vi "EMV Check All History to Cold Water Supply Temp.vi"(4 "T7_DELTA_FLOW_THRESHOLD":dbl, 6 "Cold Water Supply Temperature":dbl, 8 "error in (no error)":errorcluster, 11 "Current T7 Temperatures":dbl[](array[numeric])) -> (0 "error out":errorcluster, 5 "All History Is Near Supply Temp (T) = Flowing":bool)   [LabVIEW 2020]
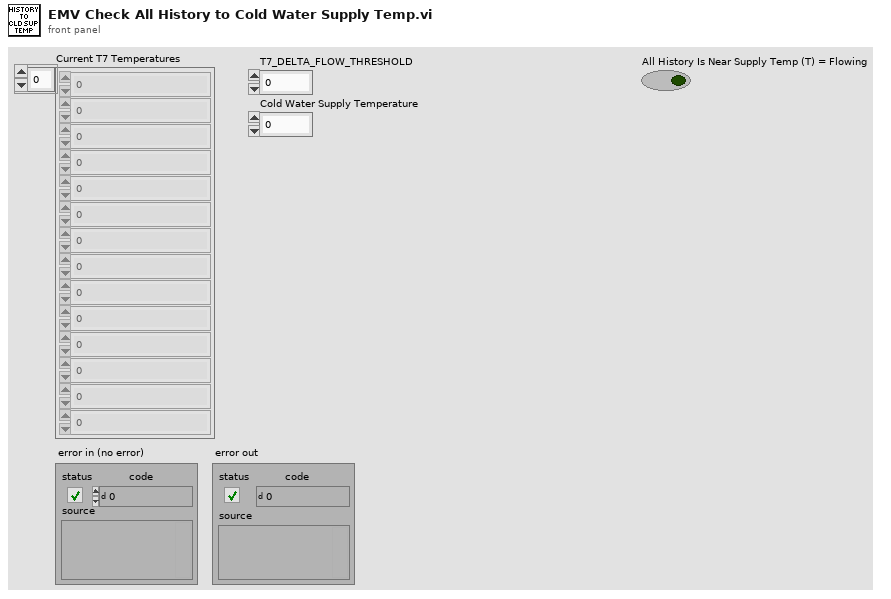
[diagram p1: front panel]
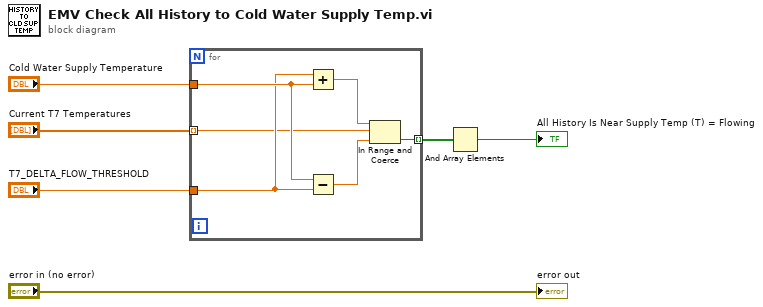
[diagram p0: block diagram]
diagram:
  n1 = for {
    tunnel: "Cold Water Supply Temperature" -> [w11]
    tunnel: "T7_DELTA_FLOW_THRESHOLD" -> [w10]
    tunnel: "Current T7 Temperatures" -> [w8] mode=indexing
    tunnel: [w7] -> w5 mode=indexing
    n2 = Add(x=w10, y=w11) -> (x+y=w12:dbl)
    n3 = Subtract(x=w11, y=w10) -> (x-y=w9:dbl)
    n4 = In Range and Coerce(upper limit=w12, x=w8, lower limit=w9) -> (In Range?=w7:bool)  [unwired: 1 out]
  }
  n5 = And Array Elements(Boolean array=w5) -> (logical AND=→"All History Is Near Supply Temp (T) = Flowing":bool)
  "error out" <- "error in (no error)"
